vi "Actor Core.vi"(8 "error in":errorcluster, 11 "CS++MotorGUI.lvclass":refnum<class "CS++MotorGui.lvclass">) -> (0 "Error Out":errorcluster, 3 "Actor out":refnum<class "Actor.lvclass">)   [LabVIEW 2015, in "CS++MotorGui.lvlib" / "CS++MotorGui.lvclass"]
doc: "(<B>Filename</B>: Actor Framework.lvlib:Actor.lvclass:Actor Core.vi)\n\nReceives messages to the actor, reacts to them, and initiates any error handling that may shut the actor down.\n\nDescendant classes may override this VI to append parallel tasks for the actor to complete while it handles messages. Overrides use the Call Parent Method node."
uses:
  CS++MotorGui.lvclass
  <vilib>/ActorFramework/Actor/Actor.lvclass
  CSPP_Core/Actors/CS++BaseActor/CS++BaseActor.lvclass/CS++BaseActor.ctl
  CSPP_Core/Actors/CS++GUIActor/CS++GUIActor.lvclass/CS++GUIActor.ctl
  CSPP_Core/Classes/CS++ProcessVariables/ProcessVariable/PV.lvclass/PV.ctl
  <vilib>/ActorFramework/Actor/Actor.lvclass/Actor.ctl
  <vilib>/ActorFramework/Message Enqueuer/Message Enqueuer.lvclass/Message Enqueuer.ctl
  CSPP_Core/Actors/CS++BaseActor/Read Object Name.vi
  CSPP_Core/Actors/CS++BaseActor/Read CS++Factory.vi
  CSPP_Core/Actors/CS++GUIActor/Read Associated Actor Name.vi
  CSPP_Core/Classes/CS++ProcessVariables/ProcessVariable/Read Data.vi
  CSPP_Core/Classes/CS++ProcessVariables/ProcessVariable/Read Timestamp.vi
  CSPP_Core/Classes/CS++ProcessVariables/ProcessVariable/Read Name.vi
  CSPP_Core/Actors/CS++GUIActor/Read Stop-Event.vi
  CSPP_Core/Actors/CS++GUIActor/Read PV-Update.vi
  CSPP_Core/Actors/CS++GUIActor/Read Associated Proxy Actor Enqueuer.vi
  <vilib>/ActorFramework/Message Enqueuer/Init from Existing Queue.vi
  <vilib>/ActorFramework/Message Enqueuer/Enqueue.vi
  <vilib>/ActorFramework/Message Priority Queue/Priority Enqueue.vi
  CSPP_Core/Classes/CS++ProcessVariables/PVConnection/PVConnection.lvclass
  CSPP_Core/Classes/CS++BaseClasses/Factory/CS++Factory.lvclass
  CSPP_Core/Classes/CS++ProcessVariables/ProcessVariable/PV.lvclass
  <vilib>/ActorFramework/Message Enqueuer/Message Enqueuer.lvclass
  <vilib>/ActorFramework/Stop Msg/Stop Msg.lvclass
  CSPP_Core/Actors/CS++DeviceGUIActor/CS++DeviceGUIActor.lvclass
  CSPP_Core/Actors/CS++GUIActor/CS++GUIActor.lvclass
  CSPP_Core/Actors/CS++BaseActor/CS++BaseActor.lvclass
  CSPP_Core/Libraries/Utilities/CS++Utilities.lvlib
panel:
  in  "Tab Control":enum32{"Info", "Control"}(tab)
  out "Last Update":timestamp
  out "Associated Device Actor":string
  out "Resource Name":string
  out "Self-Test Result Message":string
  out "Self-Test Result Code":i32
  out "Firmware Revision":string
  out "Driver Revision":string
  in  "SP2Pos":bool
  in  "Pos2SP":bool
  in  "Current File":path
  in  "Move Rel Button":bool
  in  "Save Button":bool
  in  "Load Button":bool
  in  "ManualPos":dbl
  in  "Stop All Button":bool
  in  "SetPosMode":u16(ring) items=["Manual"]
  in  "Reference Button":bool
  in  "Stop Button":bool
  in  "Move Button":bool
  in  "Axes List":i32(listbox)
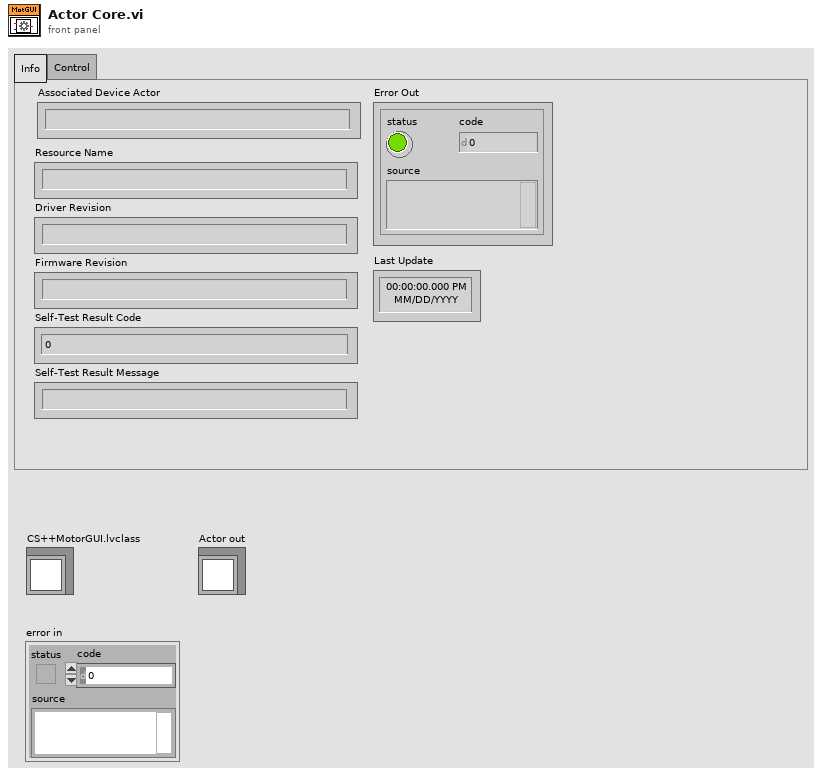
[diagram p1: front panel]
types:
  T1 = enum32{"Invalid", "Standard", "Closed", "Hidden", "Minimized", "Maximized"}
  T2 = cluster{cluster{"LogicalPosition":string, "SetPosition":dbl}[]}
  T3 = enum16{"open", "replace", "create", "open or create", "replace or create", "replace or create with confirmation"}
  T4 = cluster{cluster{"LogicalPosition":string, "SetPosition":dbl}[]}[]
  T5 = cluster{"LogicalPosition":string, "SetPosition":dbl}[]
  T6 = cluster{"LogicalPosition":string, "SetPosition":dbl}
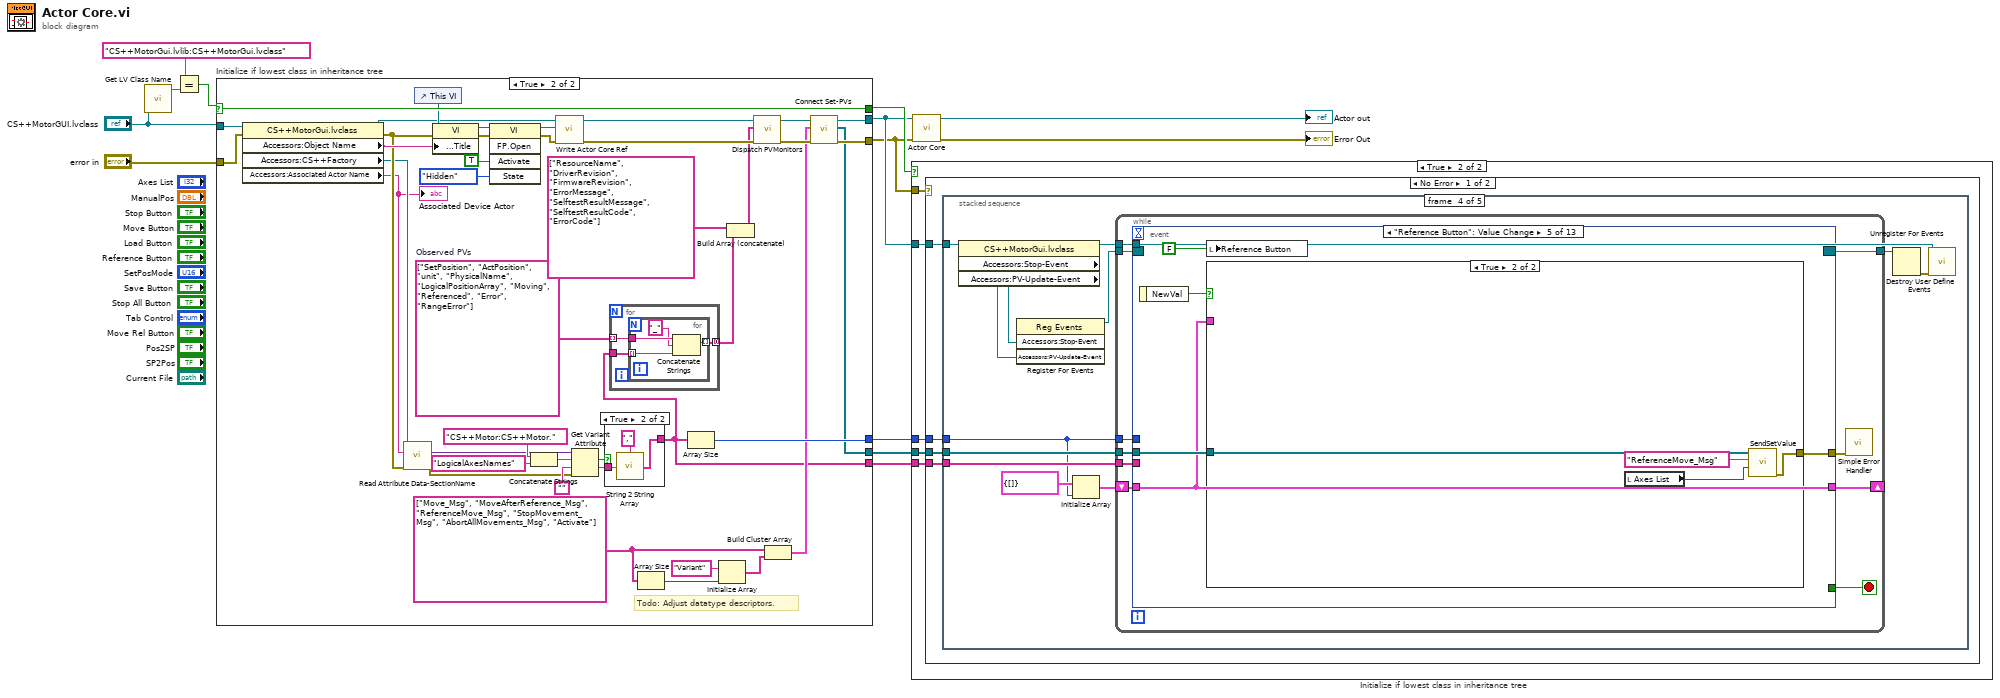
[diagram p0: block diagram]
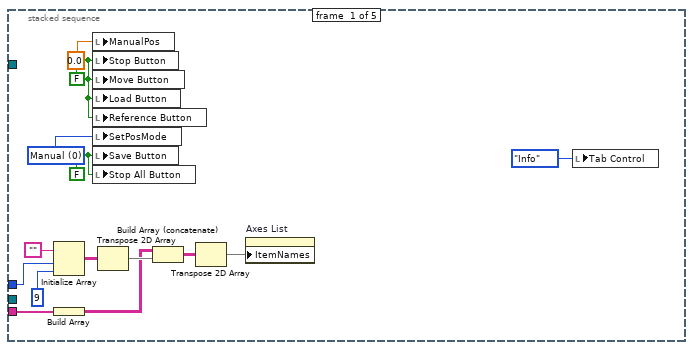
[diagram p5: hidden frame]
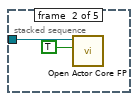
[diagram p6: hidden frame]
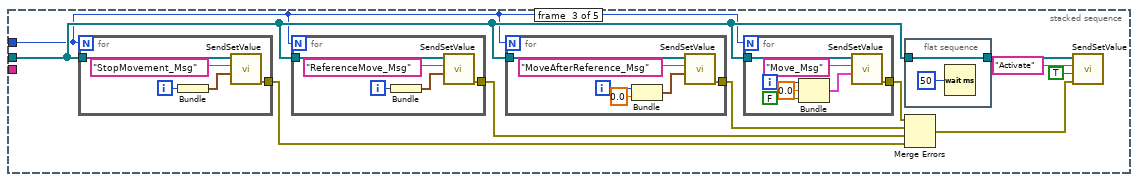
[diagram p7: hidden frame]
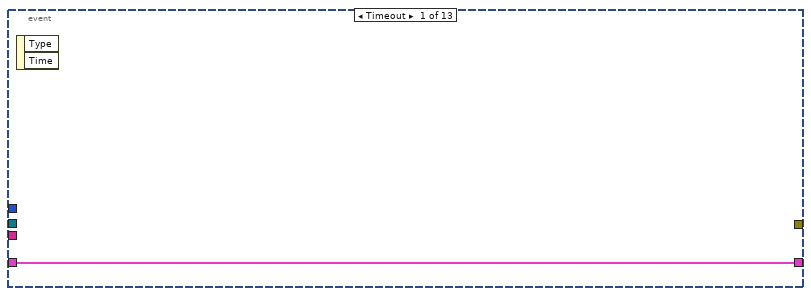
[diagram p8: hidden frame]
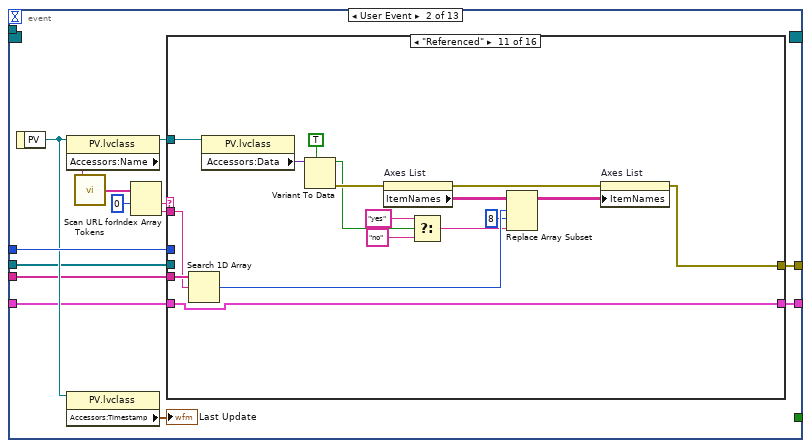
[diagram p9: hidden frame]
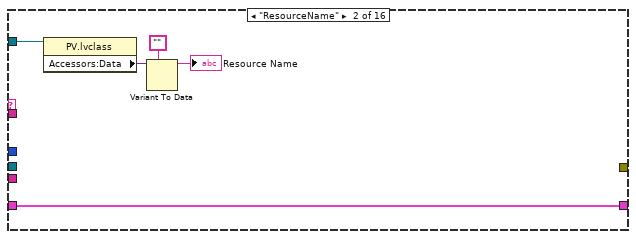
[diagram p11: hidden frame]
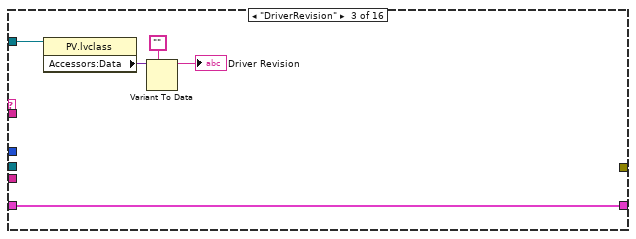
[diagram p12: hidden frame]
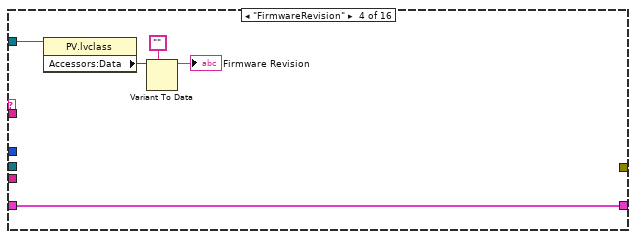
[diagram p13: hidden frame]
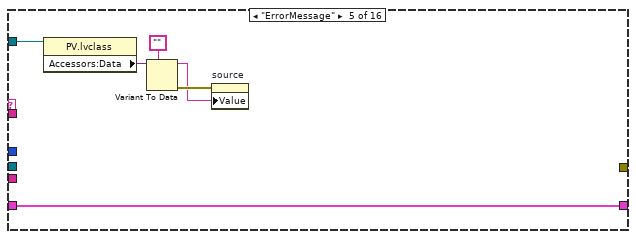
[diagram p14: hidden frame]
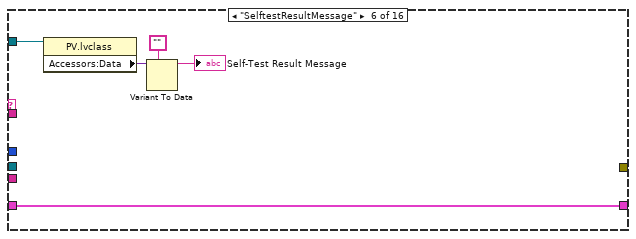
[diagram p15: hidden frame]
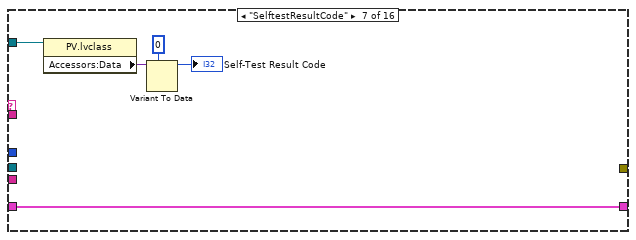
[diagram p16: hidden frame]
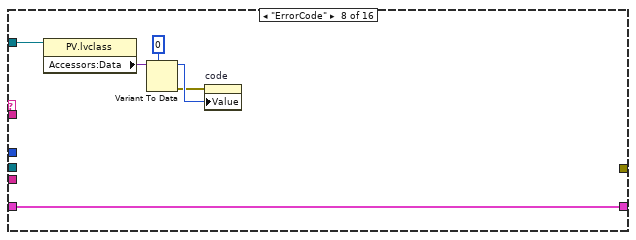
[diagram p17: hidden frame]
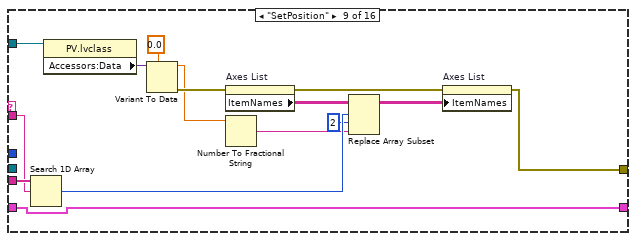
[diagram p18: hidden frame]
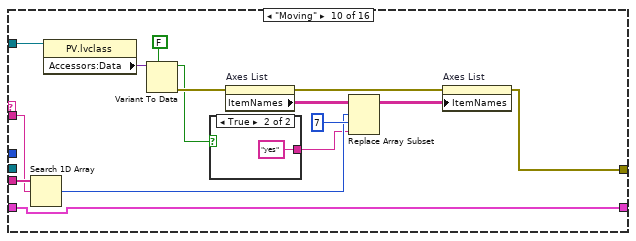
[diagram p19: hidden frame]
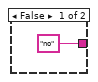
[diagram p20: hidden frame]
diagram:
  n1 = call <vilib>:"Get LV Class Name.vi"("object"="CS++MotorGUI.lvclass") -> ("class name"=w13:string)  [unwired: 9 in, 1 out]
  n2 = Equal?(x="CS++MotorGui.lvlib:CS++MotorGui.lvclass" ("class name"), y=w13) -> (x = y?=w11:bool)
  n3 = case "Initialize if lowest class in inheritance tree" shown="True" w11 {
    selector: w11 -> [w14 w57]
    tunnel: [w15 w27] -> w8
    tunnel: "error in" -> [w15 w38]
    tunnel: [w16 w28] -> w9
    tunnel: "CS++MotorGUI.lvclass" -> [w16 w39]
    tunnel: [w14 w57] -> w10
    tunnel: [_ w34] -> w7
    tunnel: [_ w18] -> w6
    tunnel: [_ w25] -> w5
    frame False {
    }
    frame True {
      w24 = string[] ["Move_Msg", "MoveAfterReference_Msg", "ReferenceMove_Msg", "StopMovement_Msg", "AbortAllMovements_Msg", "Activate"]
      w33 = string[] ["SetPosition", "ActPosition", "unit", "PhysicalName", "LogicalPositionArray", "Moving", "Referenced", "Error", "RangeError"]  # Observed PVs
      # "Todo: Adjust datatype descriptors."
      n4 = property class="CS++MotorGui.lvclass"(reference=w39, error in=w38) -> (reference out=w43:refnum<class "CS++MotorGui.lvclass">, error out=w37:errorcluster, "Accessors:Object Name"=w42:string, "Accessors:CS++Factory"=w30:refnum<class "CS++Factory.lvclass">, "Accessors:Associated Actor Name"=w17:string)
      "Associated Device Actor" <- w17
      n5 = call-dynamic "Read Attribute Data-SectionName.vi"("error in (no error)"=w37, "Object Name"=w17, "CS++Factory in"=w30) -> ("error out"=w35:errorcluster, "Attribute Data"=w36:variant)  [unwired: 6 in, 1 out]
      n6 = control-ref of="This VI"() -> (w46:refnum<vi>)
      n7 = property class="VI"(reference=w46, error in=w37, "Front Panel.Title"=w42) -> (reference out=w45:refnum<vi>, error out=w44:errorcluster)
      n8 = invoke class="VI" method="FP.Open"(reference=w45, error in=w44, "Activate"=TRUE ("Activate?"), "State"=T1."Hidden") -> (reference out=w48:refnum<vi>, error out=w47:errorcluster)  [unwired: 1 in, 3 out]
      n9 = Concatenate Strings("CS++Motor:CS++Motor.", "LogicalAxesNames" ("string")) -> (w55:string)
      n10 = call "Write Actor Core Ref.vi"("error in (no error)"=w47, "Actor Core Ref"=w48, "CS++BaseActor in"=w43) -> ("error out"=w40:errorcluster, "CS++BaseActor out"=w41:refnum<class "CS++MotorGui.lvclass">)  [unwired: 7 in]
      n11 = Get Variant Attribute(Variant=w36, name=w55, default value (empty Variant)="", error in=w35) -> (found=w52:bool, value=w53:string)  [unwired: 2 out]
      n12 = case shown="True" w52 {
        tunnel: w53 -> [_ w67]
        tunnel: [_ w65] -> w18
        frame False {
        }
        frame True {
          n13 = call "String 2 String Array.vi"("String"=w67, "Delimiter (\",\")"="," ("Delimiter (\",\")")) -> ("Substrings"=w65:string[])
        }
      }
      n14 = for {
        tunnel: w33 -> [w60] mode=indexing
        tunnel: [w59] -> w19 mode=concatenating
        tunnel: w18 -> [w58]
        n15 = for {
          tunnel: w60 -> [w64]
          tunnel: [w63] -> w59 mode=indexing
          tunnel: w58 -> [w61] mode=indexing
          n16 = Concatenate Strings(w64, "_" ("string"), w61) -> (w63:string)
        }
      }
      n17 = Array Size(array=w24) -> (size(s)=w23:i32)
      n18 = Array Size(array=w18) -> (size(s)=w34:i32)
      n19 = Initialize Array("Variant", w23) -> (w20:string[])
      n20 = Build Array (concatenate)(string[] ["ResourceName", "DriverRevision", "FirmwareRevision", "ErrorMessage", "SelftestResultMessage", "SelftestResultCode", "ErrorCode"], w19) -> (w32:string[])
      n21 = call "Dispatch PVMonitors.vi"("Error In"=w40, "PV Names (empty)"=w32, "CS++GUIActor in"=w41) -> ("Error Out"=w26:errorcluster, "CS++GUIActor out"=w29:refnum<class "CS++MotorGui.lvclass">)  [unwired: 7 in]
      n22 = Build Cluster Array(w24, w20) -> (w21:cluster{string, string}[])
      n23 = call "Connect Set-PVs.vi"("Error In"=w26, "Set-Messages"=w21, "CS++GUIActor in"=w29) -> ("Error Out"=w27:errorcluster, "PVConnections"=w25:refnum<class "PVConnection.lvclass">[], "CS++GUIActor out"=w28:refnum<class "CS++MotorGui.lvclass">)  [unwired: 6 in]
    }
  }
  n24 = case "Initialize if lowest class in inheritance tree" shown="True" w10 {
    tunnel: w8 -> [_ w72]
    tunnel: w9 -> [_ w71]
    tunnel: w7 -> [_ w70]
    tunnel: w6 -> [_ w69]
    tunnel: w5 -> [_ w68]
    frame False {
    }
    frame True {
      n25 = case shown="No Error" w72 {
        tunnel: w71 -> [w76 _]
        tunnel: w70 -> [w75 _]
        tunnel: w69 -> [w74 _]
        tunnel: w68 -> [w73 _]
        frame No Error {
          n26 = stacked-sequence {
            tunnel: w76 -> [_ w91 _ w136 w589]
            tunnel: w75 -> [w81 _ w93 w128 _]
            tunnel: w74 -> [w85 _ _ w139 _]
            tunnel: w73 -> [_ _ w95 w129 w587]
            frame #0 {
              w89 = u16 0 items=["Manual"] ("SetPosMode")
              w88 = FALSE ("Save Button")
              w87 = FALSE ("Stop Button")
              n27 = Initialize Array("", w81, 9 ("dimension size")) -> (w83:string[][])
              n28 = Build Array(w85) -> (w78:string[][])
              n29 = local write "ManualPos"(0.0 ("ManualPos")) -> ()
              n30 = local write "Stop Button"(w87) -> ()
              n31 = local write "Move Button"(w87) -> ()
              n32 = local write "Load Button"(w87) -> ()
              n33 = local write "Reference Button"(w87) -> ()
              n34 = local write "SetPosMode"(w89) -> ()
              n35 = local write "Save Button"(w88) -> ()
              n36 = local write "Stop All Button"(w88) -> ()
              n37 = Transpose 2D Array(2D array=w83) -> (transposed array=w79:string[][])
              n38 = Build Array (concatenate)(w78, w79) -> (w77:string[][])
              n39 = Transpose 2D Array(2D array=w77) -> (transposed array=w84:string[][])
              n40 = property on="Axes List" class="MCListbox (strict)"("ItemNames"=w84) -> ()  [unwired: 2 in, 2 out]
              n41 = local write "Tab Control"(enum32{"Info", "Control"}."Info" ("Tab Control")) -> ()
            }
            frame #1 {
              n42 = call "Open Actor Core FP.vi"("Open FP (F)"=TRUE, "CS++BaseActor in"=w91) -> ()  [unwired: 8 in, 2 out]
            }
            frame #2 {
              n43 = for {
                N: w93 -> [_]
                tunnel: w95 -> [w104]
                tunnel: [w103] -> w94
                i -> [w105]
                n44 = Bundle(w105) -> (w107:cluster{i32})  [unwired: 1 in]
                n45 = call "SendSetValue.vi"("Data"=w107, "PVName"="StopMovement_Msg", "PVConnections"=w104) -> ("error out"=w103:errorcluster)  [unwired: 7 in, 1 out]
              }
              n46 = for {
                N: w93 -> [_]
                tunnel: w95 -> [w109]
                tunnel: [w108] -> w96
                i -> [w110]
                n47 = Bundle(w110) -> (w112:cluster{i32})  [unwired: 1 in]
                n48 = call "SendSetValue.vi"("Data"=w112, "PVName"="ReferenceMove_Msg", "PVConnections"=w109) -> ("error out"=w108:errorcluster)  [unwired: 7 in, 1 out]
              }
              n49 = for {
                N: w93 -> [_]
                tunnel: w95 -> [w114]
                tunnel: [w113] -> w97
                i -> [w116]
                n50 = Bundle(w116, 0.0) -> (w118:cluster{i32, dbl})  [unwired: 1 in]
                n51 = call "SendSetValue.vi"("Data"=w118, "PVName"="MoveAfterReference_Msg", "PVConnections"=w114) -> ("error out"=w113:errorcluster)  [unwired: 7 in, 1 out]
              }
              n52 = for {
                N: w93 -> [_]
                tunnel: w95 -> [w120]
                tunnel: [w119] -> w99
                i -> [w123]
                n53 = Bundle(w123, 0.0, FALSE) -> (w125:cluster{i32, dbl, bool})  [unwired: 1 in]
                n54 = call "SendSetValue.vi"("Data"=w125, "PVName"="Move_Msg", "PVConnections"=w120) -> ("error out"=w119:errorcluster)  [unwired: 7 in, 1 out]
              }
              n55 = flat-sequence {
                tunnel: w95 -> [w126]
                tunnel: [w126] -> w100
                frame #0 {
                  n56 = Wait (ms)(milliseconds to wait=u32 50) -> ()  [unwired: 1 out]
                }
              }
              n57 = Merge Errors(w99, w97, w96, w94) -> (w98:errorcluster)
              n58 = call "SendSetValue.vi"("error in (no error)"=w98, "Data"=TRUE, "PVName"="Activate", "PVConnections"=w100) -> ()  [unwired: 6 in, 2 out]
            }
            frame #3 {
              n59 = property class="CS++MotorGui.lvclass"(reference=w136) -> (reference out=w135:refnum<class "CS++MotorGui.lvclass">, "Accessors:Stop-Event"=w133:refnum<user-event>, "Accessors:PV-Update-Event"=w132:refnum<user-event>)  [unwired: 1 in, 1 out]
              n60 = register-events(w133, w132) -> (reference out=w134:refnum<event-registration>)  [unwired: 2 in, 1 out]
              n61 = Initialize Array(T2 {[]}, w128) -> (w131:T4)
              n62 = while {
                tunnel: w134 -> [w149]
                tunnel: w135 -> [w148]
                tunnel: [w146] -> w138
                tunnel: w128 -> [w144]
                tunnel: w139 -> [w143]
                tunnel: w129 -> [w142]
                shift-right: [w140] -> _
                shift-left: w131 -> [w141]
                stop <- w147 stop-if-true
                n63 = event shown="[4] \"Reference Button\": Value Change" {
                  selector: w149 -> [_ _ _ _ _ _ _ _ _ _ _ _ _]
                  dyn-events: [_ _ _ _ _ _ _ _ _ _ _ _ _] -> w146
                  timeout: _ -> [_ _ _ _ _ _ _ _ _ _ _ _ _]
                  tunnel: w148 -> [_ _ _ _ _ _ _ _ _ _ _ w576 w582]
                  tunnel: [_ _ _ _ _ _ _ _ _ _ _ TRUE ("Stop") TRUE ("Stop")] -> w147
                  tunnel: [_ w161 w362 w387 w413 w422 w432 w440 w468 w517 w543 _ _] -> w145
                  tunnel: w144 -> [_ w160 _ _ _ _ w429 _ _ _ _ _ _]
                  tunnel: w143 -> [_ w153 _ _ _ _ _ _ _ _ _ _ _]
                  tunnel: w142 -> [_ w154 w363 w388 w414 w423 w433 _ _ _ w542 _ _]
                  tunnel: w141 -> [w150 w152 w361 w386 w412 w421 w431 w441 w469 w518 w544 w574 w580]
                  tunnel: [w150 w151 w361 w386 w412 w421 w431 w441 w469 w518 w544 w574 w580] -> w140
                  event Timeout {
                    n64 = event-data() -> ()  [unwired: 1 in, 2 out]
                  }
                  event User Event {
                    n65 = event-data() -> ("PV"=w156:refnum<class "PV.lvclass">)  [unwired: 1 in]
                    n66 = property class="PV.lvclass"(reference=w156) -> (reference out=w158:refnum<class "PV.lvclass">, "Accessors:Name"=w157:string)  [unwired: 1 in, 1 out]
                    n67 = property class="PV.lvclass"(reference=w156) -> ("Accessors:Timestamp"=→"Last Update":timestamp)  [unwired: 1 in, 2 out]
                    n68 = call "Scan URL for Tokens.vi"("URL"=w157) -> ("Tokens"=w163:string[])
                    n69 = Index Array(array=w163, index #1=0 ("index")) -> (element #1=w162:string, element #2=w159:string)  [unwired: 1 in]
                    n70 = case shown="\"Referenced\"" w162 {
                      tunnel: w158 -> [_ w168 w173 w178 w184 w189 w194 w200 w216 w231 w250 w268 w279 w317 w331 w348]
                      tunnel: [_ _ _ _ _ _ _ _ w211 w226 w245 w263 w285 w312 w326 w344] -> w161
                      tunnel: w160 -> [_ _ _ _ _ _ _ _ _ _ _ _ _ _ _ _]
                      tunnel: w159 -> [_ _ _ _ _ _ _ _ w209 w224 w243 w261 w283 w310 w324 w346]
                      tunnel: w154 -> [_ _ _ _ _ _ _ _ _ _ _ _ _ _ _ _]
                      tunnel: w153 -> [_ _ _ _ _ _ _ _ w210 w225 w244 w262 w284 w311 w325 w347]
                      tunnel: w152 -> [w165 w166 w171 w176 w181 w187 w192 w197 w203 w222 w239 w258 w278 w305 w319 w342]
                      tunnel: [w165 w166 w171 w176 w181 w187 w192 w197 w203 w222 w239 w258 w278 w305 w319 w341] -> w151
                      frame Default {
                      }
                      frame "ResourceName" {
                        n71 = property class="PV.lvclass"(reference=w168) -> ("Accessors:Data"=w170:variant)  [unwired: 1 in, 2 out]
                        n72 = Variant To Data(type="", Variant=w170) -> (data=→"Resource Name":string)  [unwired: 1 in, 1 out]
                      }
                      frame "DriverRevision" {
                        n73 = property class="PV.lvclass"(reference=w173) -> ("Accessors:Data"=w175:variant)  [unwired: 1 in, 2 out]
                        n74 = Variant To Data(type="", Variant=w175) -> (data=→"Driver Revision":string)  [unwired: 1 in, 1 out]
                      }
                      frame "FirmwareRevision" {
                        n75 = property class="PV.lvclass"(reference=w178) -> ("Accessors:Data"=w180:variant)  [unwired: 1 in, 2 out]
                        n76 = Variant To Data(type="", Variant=w180) -> (data=→"Firmware Revision":string)  [unwired: 1 in, 1 out]
                      }
                      frame "ErrorMessage" {
                        n77 = property class="PV.lvclass"(reference=w184) -> ("Accessors:Data"=w186:variant)  [unwired: 1 in, 2 out]
                        n78 = Variant To Data(type="", Variant=w186) -> (data=w182:string, error out=w183:errorcluster)  [unwired: 1 in]
                        n79 = property on="source" class="Str"(error in=w183, "Value"=w182) -> ()  [unwired: 1 in, 2 out]
                      }
                      frame "SelftestResultMessage" {
                        n80 = property class="PV.lvclass"(reference=w189) -> ("Accessors:Data"=w191:variant)  [unwired: 1 in, 2 out]
                        n81 = Variant To Data(type="", Variant=w191) -> (data=→"Self-Test Result Message":string)  [unwired: 1 in, 1 out]
                      }
                      frame "SelftestResultCode" {
                        n82 = property class="PV.lvclass"(reference=w194) -> ("Accessors:Data"=w196:variant)  [unwired: 1 in, 2 out]
                        n83 = Variant To Data(type=0, Variant=w196) -> (data=→"Self-Test Result Code":i32)  [unwired: 1 in, 1 out]
                      }
                      frame "ErrorCode" {
                        n84 = property class="PV.lvclass"(reference=w200) -> ("Accessors:Data"=w202:variant)  [unwired: 1 in, 2 out]
                        n85 = Variant To Data(type=0, Variant=w202) -> (data=w199:i32, error out=w198:errorcluster)  [unwired: 1 in]
                        n86 = property on="code" class="DigNum (strict)"(error in=w198, "Value"=w199) -> ()  [unwired: 1 in, 2 out]
                      }
                      frame "SetPosition" {
                        n87 = Search 1D Array(1D array=w210, element=w209) -> (index of element=w208:i32)  [unwired: 1 in]
                        n88 = property class="PV.lvclass"(reference=w216) -> ("Accessors:Data"=w217:variant)  [unwired: 1 in, 2 out]
                        n89 = Variant To Data(type=0.0, Variant=w217) -> (data=w205:dbl, error out=w213:errorcluster)  [unwired: 1 in]
                        n90 = property on="Axes List" class="MCListbox (strict)"(error in=w213) -> (error out=w212:errorcluster, "ItemNames"=w215:string[][])  [unwired: 1 in, 1 out]
                        n91 = Number To Fractional String(number=w205) -> (F-format string=w204:string)  [unwired: 3 in]
                        n92 = Replace Array Subset(array=w215, new element=w204, index (row)=w208, index (col)=2 ("disabled index (col)")) -> (w214:string[][])
                        n93 = property on="Axes List" class="MCListbox (strict)"(error in=w212, "ItemNames"=w214) -> (error out=w211:errorcluster)  [unwired: 1 in, 1 out]
                      }
                      frame "Moving" {
                        n94 = Search 1D Array(1D array=w225, element=w224) -> (index of element=w221:i32)  [unwired: 1 in]
                        n95 = property class="PV.lvclass"(reference=w231) -> ("Accessors:Data"=w232:variant)  [unwired: 1 in, 2 out]
                        n96 = Variant To Data(type=FALSE, Variant=w232) -> (data=w220:bool, error out=w228:errorcluster)  [unwired: 1 in]
                        n97 = case shown="True" w220 {
                          tunnel: ["no" "yes"] -> w219
                          frame False {
                          }
                          frame True {
                          }
                        }
                        n98 = property on="Axes List" class="MCListbox (strict)"(error in=w228) -> (error out=w227:errorcluster, "ItemNames"=w230:string[][])  [unwired: 1 in, 1 out]
                        n99 = Replace Array Subset(array=w230, new element=w219, index (row)=w221, index (col)=7 ("disabled index (col)")) -> (w229:string[][])
                        n100 = property on="Axes List" class="MCListbox (strict)"(error in=w227, "ItemNames"=w229) -> (error out=w226:errorcluster)  [unwired: 1 in, 1 out]
                      }
                      frame "Referenced" {
                        n101 = Search 1D Array(1D array=w244, element=w243) -> (index of element=w242:i32)  [unwired: 1 in]
                        n102 = property class="PV.lvclass"(reference=w250) -> ("Accessors:Data"=w251:variant)  [unwired: 1 in, 2 out]
                        n103 = Variant To Data(type=TRUE, Variant=w251) -> (data=w237:bool, error out=w247:errorcluster)  [unwired: 1 in]
                        n104 = property on="Axes List" class="MCListbox (strict)"(error in=w247) -> (error out=w246:errorcluster, "ItemNames"=w249:string[][])  [unwired: 1 in, 1 out]
                        n105 = Select(t="yes", s=w237, f="no") -> (s? t:f=w238:string)
                        n106 = Replace Array Subset(array=w249, new element=w238, index (row)=w242, index (col)=8 ("disabled index (col)")) -> (w248:string[][])
                        n107 = property on="Axes List" class="MCListbox (strict)"(error in=w246, "ItemNames"=w248) -> (error out=w245:errorcluster)  [unwired: 1 in, 1 out]
                      }
                      frame "Error" {
                        n108 = Search 1D Array(1D array=w262, element=w261) -> (index of element=w260:i32)  [unwired: 1 in]
                        n109 = property class="PV.lvclass"(reference=w268) -> ("Accessors:Data"=w269:variant)  [unwired: 1 in, 2 out]
                        n110 = Variant To Data(type=u8 0, Variant=w269) -> (data=w253:u8, error out=w265:errorcluster)  [unwired: 1 in]
                        n111 = Not Equal To 0?(x=w253) -> (x != 0?=w252:bool)
                        n112 = property on="Axes List" class="MCListbox (strict)"(error in=w265) -> (error out=w264:errorcluster, "ItemNames"=w267:string[][])  [unwired: 1 in, 1 out]
                        n113 = Select(t="yes", s=w252, f="no") -> (s? t:f=w257:string)
                        n114 = Replace Array Subset(array=w267, new element=w257, index (row)=w260, index (col)=9 ("disabled index (col)")) -> (w266:string[][])
                        n115 = property on="Axes List" class="MCListbox (strict)"(error in=w264, "ItemNames"=w266) -> (error out=w263:errorcluster)  [unwired: 1 in, 1 out]
                      }
                      frame "ActPosition" {
                        n116 = Search 1D Array(1D array=w284, element=w283) -> (index of element=w270:i32)  [unwired: 1 in]
                        n117 = property class="PV.lvclass"(reference=w279) -> ("Accessors:Data"=w289:variant)  [unwired: 1 in, 2 out]
                        n118 = Variant To Data(type=0.0, Variant=w289) -> (data=w275:dbl, error out=w287:errorcluster)  [unwired: 1 in]
                        n119 = property on="Axes List" class="MCListbox (strict)"(error in=w287) -> (error out=w286:errorcluster, "ItemNames"=w288:string[][])  [unwired: 1 in, 1 out]
                        n120 = Number To Fractional String(number=w275) -> (F-format string=w280:string)  [unwired: 3 in]
                        n121 = Index Array(array=w278, index=w270) -> (element=w277:T2)
                        n122 = Unbundle(w277) -> (w276:T5)
                        n123 = for {
                          tunnel: w276 -> [w304] mode=indexing
                          tunnel: w275 -> [w302]
                          tunnel: [w301] -> w271
                          tunnel: [w300] -> w274
                          stop <- w300 stop-if-true
                          n124 = Unbundle(w304) -> ("LogicalPosition"=w301:string, "SetPosition"=w303:dbl)
                          n125 = Equal?(x=w302, y=w303) -> (x = y?=w300:bool)
                        }
                        n126 = Replace Array Subset(array=w288, new element=w280, index (row)=w270, index (col)=3 ("disabled index (col)")) -> (w273:string[][])
                        n127 = case shown="False" w274 {
                          tunnel: w273 -> [w293 w298]
                          tunnel: [w292 w297] -> w272
                          tunnel: w271 -> [_ w295]
                          tunnel: w270 -> [w291 w296]
                          frame False {
                            n128 = Replace Array Subset(array=w293, new element="", index (row)=w291, index (col)=4 ("disabled index (col)")) -> (w292:string[][])
                          }
                          frame True {
                            n129 = Replace Array Subset(array=w298, new element=w295, index (row)=w296, index (col)=4 ("disabled index (col)")) -> (w297:string[][])
                          }
                        }
                        n130 = property on="Axes List" class="MCListbox (strict)"(error in=w286, "ItemNames"=w272) -> (error out=w285:errorcluster)  [unwired: 1 in, 1 out]
                      }
                      frame "PhysicalName" {
                        n131 = Search 1D Array(1D array=w311, element=w310) -> (index of element=w309:i32)  [unwired: 1 in]
                        n132 = property class="PV.lvclass"(reference=w317) -> ("Accessors:Data"=w318:variant)  [unwired: 1 in, 2 out]
                        n133 = Variant To Data(type="", Variant=w318) -> (data=w306:string, error out=w314:errorcluster)  [unwired: 1 in]
                        n134 = property on="Axes List" class="MCListbox (strict)"(error in=w314) -> (error out=w313:errorcluster, "ItemNames"=w316:string[][])  [unwired: 1 in, 1 out]
                        n135 = Replace Array Subset(array=w316, new element=w306, index (row)=w309, index (col)=1 ("disabled index (col)")) -> (w315:string[][])
                        n136 = property on="Axes List" class="MCListbox (strict)"(error in=w313, "ItemNames"=w315) -> (error out=w312:errorcluster)  [unwired: 1 in, 1 out]
                      }
                      frame "unit" {
                        n137 = Search 1D Array(1D array=w325, element=w324) -> (index of element=w323:i32)  [unwired: 1 in]
                        n138 = property class="PV.lvclass"(reference=w331) -> ("Accessors:Data"=w332:variant)  [unwired: 1 in, 2 out]
                        n139 = Variant To Data(type="", Variant=w332) -> (data=w320:string, error out=w328:errorcluster)  [unwired: 1 in]
                        n140 = property on="Axes List" class="MCListbox (strict)"(error in=w328) -> (error out=w327:errorcluster, "ItemNames"=w330:string[][])  [unwired: 1 in, 1 out]
                        n141 = Replace Array Subset(array=w330, new element=w320, index (row)=w323, index (col)=6 ("disabled index (col)")) -> (w329:string[][])
                        n142 = property on="Axes List" class="MCListbox (strict)"(error in=w327, "ItemNames"=w329) -> (error out=w326:errorcluster)  [unwired: 1 in, 1 out]
                      }
                      frame "LogicalPositionArray" {
                        n143 = Search 1D Array(1D array=w347, element=w346) -> (index of element=w338:i32)  [unwired: 1 in]
                        n144 = property class="PV.lvclass"(reference=w348) -> ("Accessors:Data"=w349:variant)  [unwired: 1 in, 2 out]
                        n145 = Variant To Data(type="", Variant=w349) -> (data=w343:string, error out=w344:errorcluster)  [unwired: 1 in]
                        n146 = while {
                          tunnel: [w358] -> w339 mode=indexing
                          shift-right: [w353] -> _
                          shift-left: w343 -> [w360]
                          tunnel: [w351] -> w335 mode=indexing
                          stop <- w352 stop-if-true
                          n147 = Match Pattern(string=w360, regular expression="/") -> (before substring=w351:string, after substring=w356:string)  [unwired: 1 in, 2 out]
                          n148 = Match Pattern(string=w356, regular expression="/") -> (before substring=w354:string, after substring=w353:string)  [unwired: 1 in, 2 out]
                          n149 = Fract/Exp String To Number(string=w354) -> (number=w355:dbl)  [unwired: 3 in, 1 out]
                          n150 = Empty String/Path?(string/path=w353) -> (empty?=w352:bool)
                          n151 = Bundle(w351, w355) -> (w358:cluster{string, dbl})  [unwired: 1 in]
                        }
                        n152 = Build Array (concatenate)("Manual", w335) -> (w333:string[])
                        n153 = local read "Axes List"() -> (w337:i32)
                        n154 = Bundle(w339) -> (w340:cluster{cluster{string, dbl}[]})  [unwired: 1 in]
                        n155 = Replace Array Subset(array=w342, new element=w340, index=w338) -> (w341:T4)
                        n156 = Equal?(x=w338, y=w337) -> (x = y?=w336:bool)
                        n157 = case shown="True" w336 {
                          tunnel: w333 -> [_ w350]
                          frame False {
                          }
                          frame True {
                            n158 = property on="SetPosMode" class="Ring (strict)"("Strings []"=w350) -> ()  [unwired: 2 in, 2 out]
                          }
                        }
                      }
                    }
                  }
                  event "Move Button": Value Change {
                    n159 = event-data() -> ("NewVal"=w365:bool)  [unwired: 1 in]
                    n160 = local write "Move Button"(FALSE ("Move Button")) -> ()
                    n161 = case shown="True" w365 {
                      tunnel: w363 -> [_ w368]
                      tunnel: [_ w369] -> w362
                      tunnel: w361 -> [_ w374]
                      frame False {
                      }
                      frame True {
                        n162 = local read "SetPosMode"() -> (w375:u16)
                        n163 = local read "Axes List"() -> (w367:i32)
                        n164 = local read "ManualPos"() -> (w376:dbl)
                        n165 = Equal To 0?(x=w375) -> (x = 0?=w377:bool)
                        n166 = Decrement(x=w375) -> (x-1=w373:u16)
                        n167 = case shown="False" w377 {
                          tunnel: [w380 w385] -> w366
                          tunnel: w376 -> [_ w385]
                          tunnel: w374 -> [w384 _]
                          tunnel: w373 -> [w379 _]
                          tunnel: w367 -> [w378 _]
                          frame False {
                            n168 = Index Array(array=w384, index=w378) -> (element=w383:T2)
                            n169 = Unbundle(w383) -> (w382:T5)
                            n170 = Index Array(array=w382, index=w379) -> (element=w381:T6)
                            n171 = Unbundle(w381) -> ("SetPosition"=w380:dbl)  [unwired: 1 out]
                          }
                          frame True {
                          }
                        }
                        n172 = Bundle("Axes List"=w367, "ManualPos"=w366, FALSE) -> (w371:cluster{"Axes List":i32, "ManualPos":dbl, bool})  [unwired: 1 in]
                        n173 = call "SendSetValue.vi"("Data"=w371, "PVName"="Move_Msg", "PVConnections"=w368) -> ("error out"=w369:errorcluster)  [unwired: 7 in, 1 out]
                      }
                    }
                  }
                  event "Move Rel Button": Value Change {
                    n174 = event-data() -> ("NewVal"=w390:bool)  [unwired: 1 in]
                    n175 = local write "Move Rel Button"(FALSE ("Move Button")) -> ()
                    n176 = case shown="True" w390 {
                      tunnel: w388 -> [_ w393]
                      tunnel: [_ w394] -> w387
                      tunnel: w386 -> [_ w399]
                      frame False {
                      }
                      frame True {
                        n177 = local read "SetPosMode"() -> (w400:u16)
                        n178 = local read "Axes List"() -> (w392:i32)
                        n179 = local read "ManualPos"() -> (w401:dbl)
                        n180 = Equal To 0?(x=w400) -> (x = 0?=w402:bool)
                        n181 = Decrement(x=w400) -> (x-1=w398:u16)
                        n182 = case shown="False" w402 {
                          tunnel: [w405 w410] -> w391
                          tunnel: w401 -> [_ w410]
                          tunnel: w399 -> [w409 _]
                          tunnel: w398 -> [w404 _]
                          tunnel: w392 -> [w403 _]
                          frame False {
                            n183 = Index Array(array=w409, index=w403) -> (element=w408:T2)
                            n184 = Unbundle(w408) -> (w407:T5)
                            n185 = Index Array(array=w407, index=w404) -> (element=w406:T6)
                            n186 = Unbundle(w406) -> ("SetPosition"=w405:dbl)  [unwired: 1 out]
                          }
                          frame True {
                          }
                        }
                        n187 = Bundle("Axes List"=w392, "ManualPos"=w391, TRUE) -> (w396:cluster{"Axes List":i32, "ManualPos":dbl, bool})  [unwired: 1 in]
                        n188 = call "SendSetValue.vi"("Data"=w396, "PVName"="Move_Msg", "PVConnections"=w393) -> ("error out"=w394:errorcluster)  [unwired: 7 in, 1 out]
                      }
                    }
                  }
                  event "Reference Button": Value Change {
                    n189 = event-data() -> ("NewVal"=w415:bool)  [unwired: 1 in]
                    n190 = local write "Reference Button"(FALSE ("Move Button")) -> ()
                    n191 = case shown="True" w415 {
                      tunnel: w414 -> [_ w419]
                      tunnel: [_ w418] -> w413
                      tunnel: w412 -> [_ _]
                      frame False {
                      }
                      frame True {
                        n192 = local read "Axes List"() -> (w416:i32)
                        n193 = call "SendSetValue.vi"("Data"=w416, "PVName"="ReferenceMove_Msg", "PVConnections"=w419) -> ("error out"=w418:errorcluster)  [unwired: 7 in, 1 out]
                      }
                    }
                  }
                  event "Stop Button": Value Change {
                    n194 = event-data() -> ("NewVal"=w424:bool)  [unwired: 1 in]
                    n195 = local write "Stop Button"(FALSE ("Move Button")) -> ()
                    n196 = case shown="True" w424 {
                      tunnel: w423 -> [_ w428]
                      tunnel: [_ w427] -> w422
                      tunnel: w421 -> [_ _]
                      frame False {
                      }
                      frame True {
                        n197 = local read "Axes List"() -> (w425:i32)
                        n198 = call "SendSetValue.vi"("Data"=w425, "PVName"="StopMovement_Msg", "PVConnections"=w428) -> ("error out"=w427:errorcluster)  [unwired: 7 in, 1 out]
                      }
                    }
                  }
                  event "Stop All Button": Value Change {
                    n199 = event-data() -> ("NewVal"=w434:bool)  [unwired: 1 in]
                    n200 = local write "Stop All Button"(FALSE ("Move Button")) -> ()
                    n201 = case shown="True" w434 {
                      tunnel: w433 -> [_ w439]
                      tunnel: [_ w437] -> w432
                      tunnel: w431 -> [_ _]
                      tunnel: w429 -> [_ _]
                      frame False {
                      }
                      frame True {
                        n202 = call "SendSetValue.vi"("Data"=TRUE, "PVName"="AbortAllMovements_Msg", "PVConnections"=w439) -> ("error out"=w438:errorcluster)  [unwired: 7 in, 1 out]
                        n203 = Merge Errors(w438) -> (w437:errorcluster)
                      }
                    }
                  }
                  event "Save Button": Value Change {
                    n204 = event-data() -> ("NewVal"=w442:bool)  [unwired: 1 in]
                    n205 = local write "Save Button"(FALSE ("Save Button")) -> ()
                    n206 = case shown="True" w442 {
                      tunnel: [_ w457] -> w440
                      frame False {
                      }
                      frame True {
                        w449 = "|"
                        n207 = property on="Axes List" class="MCListbox (strict)"() -> (error out=w458:errorcluster, "ItemNames"=w466:string[][])  [unwired: 2 in, 1 out]
                        n208 = Index Array(array=w466, index (col) #1=0 ("disabled index (col)"), index (col) #2=1 ("index (col)"), index (col) #3=5 ("index (col)")) -> (element #1=w455:string[], element #2=w453:string[], element #3=w452:string[])  [unwired: 3 in]
                        n209 = call "String Array 2 String.vi"("Substrings"=w455, "Delimiter (\",\")"=w449) -> ("String"=w454:string)
                        n210 = call "String Array 2 String.vi"("Substrings"=w453, "Delimiter (\",\")"=w449) -> ("String"=w448:string)
                        n211 = call "String Array 2 String.vi"("Substrings"=w452, "Delimiter (\",\")"=w449) -> ("String"=w447:string)
                        n212 = Build Array(w454, w448, w447) -> (w445:string[])
                        n213 = call "String Array 2 String.vi"("Substrings"=w445, "Delimiter (\",\")"="/") -> ("String"=w446:string)
                        n214 = Open/Create/Replace File(error in=w458, operation (0:open)=T3."replace or create with confirmation", access (0:read/write)=enum16{"read/write", "read-only", "write-only"}."write-only") -> (refnum out=w460:refnum<file>, error out=w459:errorcluster)  [unwired: 3 in, 1 out]
                        n215 = Write to Text File(file (use dialog)=w460, text=w446, error in=w459) -> (refnum out=w462:refnum<file>, error out=w461:errorcluster)  [unwired: 1 in, 1 out]
                        n216 = Close File(refnum=w462, error in=w461) -> (path=w456:path, error out=w457:errorcluster)
                        n217 = local write "Current File"(w456) -> ()
                      }
                    }
                  }
                  event "Load Button": Value Change {
                    n218 = event-data() -> ("NewVal"=w470:bool)  [unwired: 1 in]
                    n219 = local write "Load Button"(FALSE ("Save Button")) -> ()
                    n220 = case shown="True" w470 {
                      tunnel: [_ w491] -> w468
                      frame False {
                      }
                      frame True {
                        w477 = "|"
                        n221 = Open/Create/Replace File(access (0:read/write)=enum16{"read/write", "read-only", "write-only"}."read-only") -> (refnum out=w494:refnum<file>, error out=w493:errorcluster)  [unwired: 5 in, 1 out]
                        n222 = Read from Text File(file (use dialog)=w494, error in=w493) -> (refnum out=w496:refnum<file>, text=w476:string, error out=w495:errorcluster)  [unwired: 2 in, 1 out]
                        n223 = call "String 2 String Array.vi"("String"=w476, "Delimiter (\",\")"="/") -> ("Substrings"=w474:string[])
                        n224 = Close File(refnum=w496, error in=w495) -> (path=w492:path, error out=w490:errorcluster)
                        n225 = property on="Axes List" class="MCListbox (strict)"(error in=w490) -> (error out=w479:errorcluster, "ItemNames"=w481:string[][])  [unwired: 1 in, 1 out]
                        n226 = local write "Current File"(w492) -> ()
                        n227 = Index Array(array=w474) -> (element #1=w473:string, element #2=w472:string, element #3=w471:string)  [unwired: 3 in]
                        n228 = call "String 2 String Array.vi"("String"=w473, "Delimiter (\",\")"=w477) -> ("Substrings"=w485:string[])
                        n229 = call "String 2 String Array.vi"("String"=w472, "Delimiter (\",\")"=w477) -> ("Substrings"=w489:string[])
                        n230 = call "String 2 String Array.vi"("String"=w471, "Delimiter (\",\")"=w477) -> ("Substrings"=w488:string[])
                        n231 = Index Array(array=w481, index (col) #1=0 ("disabled index (col)"), index (col) #2=1 ("index (col)")) -> (element #1=w487:string[], element #2=w486:string[])  [unwired: 2 in]
                        n232 = Array Size(array=w485) -> (size(s)=w484:i32)
                        n233 = for {
                          tunnel: w485 -> [w508] mode=indexing
                          tunnel: w489 -> [w507] mode=indexing
                          tunnel: w488 -> [w500] mode=indexing
                          tunnel: w487 -> [w510]
                          tunnel: w486 -> [w509]
                          shift-right: [w502] -> w482
                          shift-left: w481 -> [w503]
                          n234 = Search 1D Array(1D array=w510, element=w508) -> (index of element=w501:i32)  [unwired: 1 in]
                          n235 = Search 1D Array(1D array=w509, element=w507) -> (index of element=w506:i32)  [unwired: 1 in]
                          n236 = Equal?(x=w501, y=w506) -> (x = y?=w505:bool)
                          n237 = Greater Or Equal To 0?(x=w506) -> (x >= 0?=w504:bool)
                          n238 = And(x=w505, y=w504) -> (x .and. y?=w499:bool)
                          n239 = case shown="True" w499 {
                            tunnel: w503 -> [w511 w516]
                            tunnel: [w511 w515] -> w502
                            tunnel: w501 -> [_ w513]
                            tunnel: w500 -> [_ w512]
                            frame False {
                            }
                            frame True {
                              n240 = Replace Array Subset(array=w516, new element=w512, index (row)=w513, index (col)=5) -> (w515:string[][])
                            }
                          }
                        }
                        n241 = Not Equal To 0?(x=w484) -> (x != 0?=w483:bool)
                        n242 = Select(t=w482, s=w483, f=w481) -> (s? t:f=w480:string[][])
                        n243 = property on="Axes List" class="MCListbox (strict)"(error in=w479, "ItemNames"=w480) -> (error out=w491:errorcluster)  [unwired: 1 in, 1 out]
                      }
                    }
                  }
                  event "Pos2SP": Value Change {
                    n244 = event-data() -> ("NewVal"=w520:bool)  [unwired: 1 in]
                    n245 = local write "Pos2SP"(FALSE ("Save Button")) -> ()
                    n246 = case shown="True" w520 {
                      tunnel: w518 -> [_ w523]
                      tunnel: [_ w521] -> w517
                      frame False {
                      }
                      frame True {
                        n247 = property on="Axes List" class="MCListbox (strict)"() -> (error out=w528:errorcluster, "ItemNames"=w527:string[][])  [unwired: 2 in, 1 out]
                        n248 = Index Array(array=w527, index (col)=2 ("disabled index (col)")) -> (element=w524:string[])  [unwired: 1 in]
                        n249 = for {
                          tunnel: w524 -> [w531] mode=indexing
                          tunnel: w523 -> [w535] mode=indexing
                          tunnel: [w530] -> w522 mode=indexing
                          n250 = Unbundle(w535) -> (w534:T5)
                          n251 = for {
                            tunnel: w534 -> [w541] mode=indexing
                            tunnel: w531 -> [w539]
                            tunnel: [w537] -> w533
                            tunnel: [w536] -> w532
                            stop <- w537 stop-if-true
                            n252 = Unbundle(w541) -> ("LogicalPosition"=w536:string, "SetPosition"=w540:dbl)
                            n253 = Number To Fractional String(number=w540) -> (F-format string=w538:string)  [unwired: 3 in]
                            n254 = Equal?(x=w539, y=w538) -> (x = y?=w537:bool)
                          }
                          n255 = Select(t=w532, s=w533, f=w531) -> (s? t:f=w530:string)
                        }
                        n256 = Replace Array Subset(array=w527, new element=w522, index (col)=5 ("disabled index (col)")) -> (w526:string[][])  [unwired: 1 in]
                        n257 = property on="Axes List" class="MCListbox (strict)"(error in=w528, "ItemNames"=w526) -> (error out=w521:errorcluster)  [unwired: 1 in, 1 out]
                      }
                    }
                  }
                  event "SP2Pos": Value Change {
                    n258 = event-data() -> ("NewVal"=w546:bool)  [unwired: 1 in]
                    n259 = local write "SP2Pos"(FALSE ("Save Button")) -> ()
                    n260 = case shown="True" w546 {
                      tunnel: w544 -> [_ w550]
                      tunnel: [_ w548] -> w543
                      tunnel: w542 -> [_ w547]
                      frame False {
                      }
                      frame True {
                        n261 = property on="Axes List" class="MCListbox (strict)"() -> ("ItemNames"=w556:string[][])  [unwired: 2 in, 2 out]
                        n262 = Index Array(array=w556, index (col) #1=5 ("disabled index (col)"), index (col) #2=8 ("index (col)")) -> (element #1=w551:string[], element #2=w553:string[])  [unwired: 2 in]
                        n263 = Equal?(x=w553, y="yes") -> (x = y?=w552:bool[])
                        n264 = for {
                          tunnel: w552 -> [_] mode=indexing
                          tunnel: w551 -> [w569] mode=indexing
                          tunnel: w550 -> [w570] mode=indexing
                          tunnel: [w561] -> w549 mode=indexing
                          tunnel: w547 -> [w558]
                          i -> [w560]
                          n265 = Unbundle(w570) -> (w568:T5)
                          n266 = for {
                            tunnel: w568 -> [w573] mode=indexing
                            tunnel: [w572] -> w567 mode=indexing
                            tunnel: [w571] -> w566 mode=indexing
                            n267 = Unbundle(w573) -> ("LogicalPosition"=w572:string, "SetPosition"=w571:dbl)
                          }
                          n268 = Search 1D Array(1D array=w567, element=w569) -> (index of element=w565:i32)  [unwired: 1 in]
                          n269 = Index Array(array=w566, index=w565) -> (element=w559:dbl)
                          n270 = Bundle(w560, "SetPosition"=w559, FALSE) -> (w563:cluster{i32, "SetPosition":dbl, bool})  [unwired: 1 in]
                          n271 = call "SendSetValue.vi"("Data"=w563, "PVName"="Move_Msg", "PVConnections"=w558) -> ("error out"=w561:errorcluster)  [unwired: 7 in, 1 out]
                        }
                        n272 = Merge Errors(w549) -> (w548:errorcluster)
                      }
                    }
                  }
                  event Panel Close? {
                    n273 = event-data() -> ()  [unwired: 1 in, 1 out]
                    n274 = call <vilib>:"Read Self Enqueuer.vi"("Actor"=w576) -> ("Self Enqueuer"=w578:refnum<class "Message Enqueuer.lvclass">)  [unwired: 10 in]
                    n275 = call <vilib>:"Send Normal Stop.vi"("Message Enqueuer"=w578) -> ("error out"=w577:errorcluster)  [unwired: 10 in]
                    n276 = call <vilib>:"Simple Error Handler.vi"("error in (no error)"=w577) -> ()  [unwired: 4 in, 5 out]
                    n277 = event-data("Discard?"=TRUE) -> ()  [unwired: 1 in, 1 out]
                  }
                  event User Event {
                    n278 = event-data() -> ()  [unwired: 1 in, 5 out]
                    n279 = call <vilib>:"Read Self Enqueuer.vi"("Actor"=w582) -> ("Self Enqueuer"=w584:refnum<class "Message Enqueuer.lvclass">)  [unwired: 10 in]
                    n280 = call <vilib>:"Send Normal Stop.vi"("Message Enqueuer"=w584) -> ("error out"=w583:errorcluster)  [unwired: 10 in]
                    n281 = call <vilib>:"Simple Error Handler.vi"("error in (no error)"=w583) -> ()  [unwired: 4 in, 5 out]
                  }
                }
                n282 = call <vilib>:"Simple Error Handler.vi"("error in (no error)"=w145) -> ()  [unwired: 4 in, 5 out]
              }
              n283 = Unregister For Events(event registration refnum=w138) -> (error out=w137:errorcluster)  [unwired: 1 in]
              n284 = call-dynamic "Destroy User Define Events.vi"("error in (no error)"=w137, "CS++GUIActor in"=w135) -> ()  [unwired: 8 in, 2 out]
            }
            frame #4 {
              # "ToDo: This destroys the complete device object.\nMaybe someone only wants to close the GUI. \nBut in this case one should also be able to only \nopen the GUI without starting a second Proxy which\nwill not work (--> Object Manager)"
              n285 = for {
                tunnel: w587 -> [w599] mode=indexing
                n286 = call "Disconnect.vi"("PVConnection in"=w599) -> ()  [unwired: 9 in, 2 out]
              }
              n287 = call "Open Actor Core FP.vi"("Open FP (F)"=FALSE, "CS++BaseActor in"=w589) -> ("error out"=w585:errorcluster, "CS++BaseActor out"=w586:refnum<class "CS++MotorGui.lvclass">)  [unwired: 8 in]
              n288 = disable-structure shown="Enabled" {
                disable-tunnel: w586 -> [w594 _]
                disable-tunnel: w585 -> [w592 _]
                frame Enabled {
                  n289 = property class="CS++MotorGui.lvclass"(reference=w594, error in=w592) -> (error out=w593:errorcluster, "Accessors:Associated Proxy Actor Enqueuer"=w591:refnum<class "Message Enqueuer.lvclass">)  [unwired: 1 out]
                  n290 = call <vilib>:"Equals Not A Refnum.vi"("Message Enqueuer"=w591) -> ("Not a refnum?"=w590:bool)  [unwired: 10 in]
                  n291 = case shown="False" w590 {
                    tunnel: [w597 w598] -> _
                    tunnel: w591 -> [w596 _]
                    tunnel: w593 -> [w595 w598]
                    frame False {
                      n292 = call <vilib>:"Send Normal Stop.vi"("error in (no error)"=w595, "Message Enqueuer"=w596) -> ("error out"=w597:errorcluster)  [unwired: 9 in]
                    }
                    frame True {
                    }
                  }
                }
                frame Disabled {
                }
              }
            }
          }
        }
        frame Error {
        }
      }
    }
  }
  n293 = call-parent "Actor Core.vi"("error in"=w8, "CS++DeviceGUIActor.lvclass"=w9) -> ("Error Out"=→"Error Out":errorcluster, "Actor out"=→"Actor out":refnum<class "Actor.lvclass">)  [unwired: 8 in]
